vi "Command & Ack - Send Ack.vi"(7 "Timeout (-1)":i32=-1, 8 "error in (no error)":errorcluster, 9 "Message Data":variant, 10 "Message":string, 11 "SV B-M (Target) In":refnum<class "SV B-M (Target).lvclass">) -> (0 "error out":errorcluster, 3 "SV B-M (Target) Out":refnum<class "SV B-M (Target).lvclass">, 4 "Timeout?":bool)   [LabVIEW 2015, in "SV B-M (Target).lvclass"]
uses:
  SV B-M (Target).lvclass
  Type Defs/Message Cluster.ctl
  SV B-M (Target).lvclass/SV B-M (Target).ctl
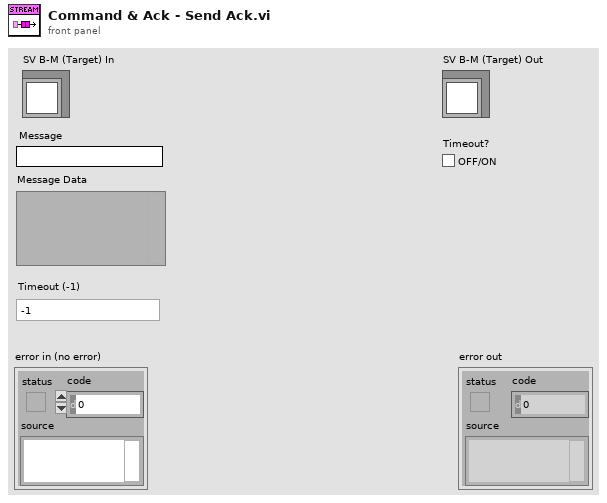
[diagram p1: front panel]
types:
  T1 = typedef "Message Cluster.ctl" = cluster{"Message":string, "Message Data":variant}
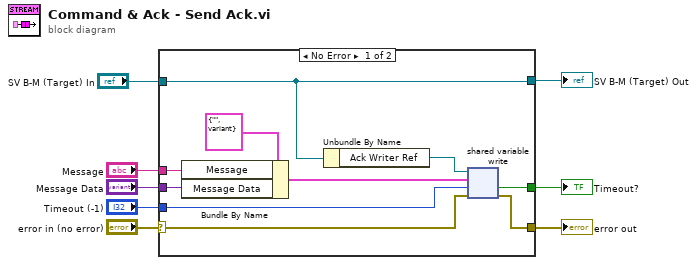
[diagram p0: block diagram]
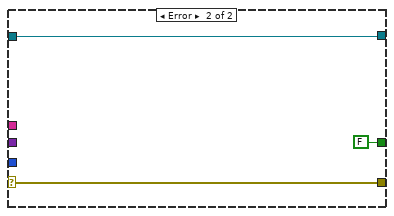
[diagram p2: hidden frame]
diagram:
  n1 = case shown="No Error" "error in (no error)" {
    selector: "error in (no error)" -> [w14 w20]
    tunnel: "SV B-M (Target) In" -> [w15 w21]
    tunnel: [w15 w21] -> w7
    tunnel: [w13 w20] -> w5
    tunnel: "Message" -> [w12 _]
    tunnel: "Message Data" -> [w11 _]
    tunnel: "Timeout (-1)" -> [w10 _]
    tunnel: [w9 FALSE] -> w1
    frame No Error {
      n2 = Bundle By Name(cluster=T1 {"Message"="", "Message Data"=variant} ("Message Cluster"), "Message"=w12, "Message Data"=w11) -> (w16:T1)
      n3 = Unbundle By Name(w15) -> ("Ack Writer Ref"=w18:refnum<k21>)
      n4 = shared-variable-write(w18, w14, w16, w10) -> (w13:errorcluster, w9:bool)  [unwired: 1 out]
    }
    frame Error {
    }
  }
  "error out" <- w5
  "SV B-M (Target) Out" <- w7
  "Timeout?" <- w1
